vi "Convert Key to String.vi"(11 "Key":u8(ring)) -> (3 "Key String":string)   [LabVIEW 2020, in "MacroAssert.lvlib" / "Keyboard Action.lvclass"]
uses:
  Keyboard Action.lvclass
  Keyboard Action.lvclass/Keyboard Action.ctl
panel:
  in  "Virtual Key":u8(ring)=65
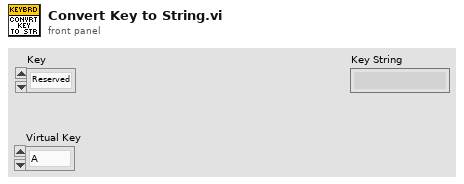
[diagram p1: front panel]
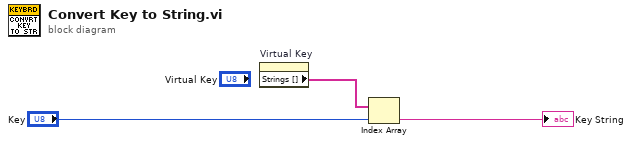
[diagram p0: block diagram]
diagram:
  n1 = property on="Virtual Key" class="Ring (strict)"() -> ("Strings []"=w3:string[])  [unwired: 2 in, 2 out]
  n2 = Index Array(array=w3, index="Key") -> (element=→"Key String":string)
